vi "Check info str.vi"(8 "error in (no error)":errorcluster, 10 "Data in":string, 11 "Motor info":T1={"Motor positions"=[0.0, 0.0], "Sensor value"=0.0, "Ens-stop state"=[FALSE, FALSE], "°/step"=[], "Motor params"={"Action"=2, "Direction motor 1"=1, "Direction motor 2"=1, "Steps motor 1"=100, "Steps motor 2"=100, "Step style motor 1"=1, "Step style motor 2"=1}} {"Motor params"."Step style motor 2" items=["", "Single", "Double", "Interleave", "Microstep"]; "Motor params"."Step style motor 1" items=["", "Single", "Double", "Interleave", "Microstep"]; "Motor params"."Direction motor 2" items=["", "Forward", "Backward"]; "Motor params"."Direction motor 1" items=["", "Forward", "Backward"]; "Motor params"."Action" items=["", "Initialize", "Move"]; "°/step" format="%#_13g"}) -> (0 "error out":errorcluster, 3 "Motor info out":T1={"Motor positions"=[0.0, 0.0], "Sensor value"=0.0, "Ens-stop state"=[FALSE, FALSE], "°/step"=[], "Motor params"={"Action"=2, "Direction motor 1"=1, "Direction motor 2"=1, "Steps motor 1"=100, "Steps motor 2"=100, "Step style motor 1"=1, "Step style motor 2"=1}} {"Motor params"."Step style motor 2" items=["", "Single", "Double", "Interleave", "Microstep"]; "Motor params"."Step style motor 1" items=["", "Single", "Double", "Interleave", "Microstep"]; "Motor params"."Direction motor 2" items=["", "Forward", "Backward"]; "Motor params"."Direction motor 1" items=["", "Forward", "Backward"]; "Motor params"."Action" items=["", "Initialize", "Move"]; "°/step" format="%#_13g"})   [LabVIEW 2020, in "Control de MaP.lvlib"]
uses:
  Control de MaP.lvlib
  Controls/Motor info.ctl
  Controls/Move motor parameters--cluster.ctl
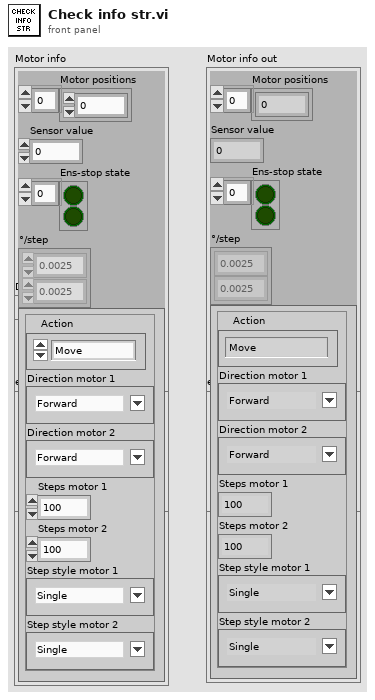
[diagram p1: front panel]
types:
  T1 = typedef "Control de MaP.lvlib/Motor info.ctl" = cluster{"Motor positions":dbl[], "Sensor value":dbl, "Ens-stop state":bool[], "°/step":dbl[], "Motor params":T2}
  T2 = typedef "Control de MaP.lvlib/Move motor parameters--cluster.ctl" = cluster{"Action":u8, "Direction motor 1":u8, "Direction motor 2":u8, "Steps motor 1":u16, "Steps motor 2":u16, "Step style motor 1":u8, "Step style motor 2":u8}
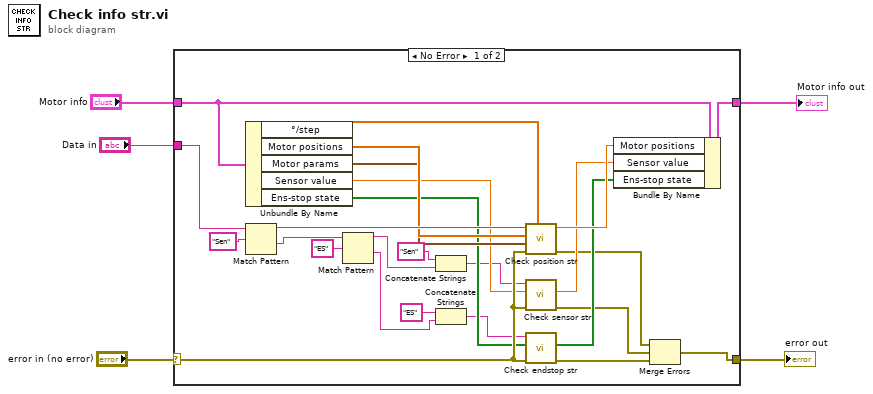
[diagram p0: block diagram]
diagram:
  n1 = case shown="No Error" "error in (no error)" {
    selector: "error in (no error)" -> [w21 w33]
    tunnel: "Data in" -> [w28 _]
    tunnel: [w17 w33] -> w3
    tunnel: "Motor info" -> [w25 w32]
    tunnel: [w15 w32] -> w1
    frame No Error {
      n2 = Unbundle By Name(w25) -> ("°/step"=w16:dbl[], "Motor positions"=w26:dbl[], "Motor params"=w14:T2, "Sensor value"=w13:dbl, "Ens-stop state"=w12:bool[])
      n3 = Match Pattern(string=w28, regular expression="Sen") -> (before substring=w27:string, after substring=w30:string)  [unwired: 1 in, 2 out]
      n4 = Match Pattern(string=w30, regular expression="ES") -> (before substring=w11:string, after substring=w7:string)  [unwired: 1 in, 2 out]
      n5 = Concatenate Strings("Sen" ("string"), w11) -> (w9:string)
      n6 = Concatenate Strings("ES" ("string"), w7) -> (w6:string)
      n7 = call "Check position str.vi"("mm/step"=w16, "error in (no error)"=w21, "Motor params"=w14, "Position in"=w26, "Recibo de Datos"=w27) -> ("error out"=w20:errorcluster, "Position out"=w24:dbl)  [unwired: 4 in, 1 out]
      n8 = call "Check sensor str.vi"("error in (no error)"=w21, "Sensor value in"=w13, "string"=w9) -> ("error out"=w19:errorcluster, "Sensor value out"=w23:dbl)  [unwired: 6 in]
      n9 = call "Check endstop str.vi"("error in (no error)"=w21, "Ens-stop state in"=w12, "Data in"=w6) -> ("error out"=w18:errorcluster, "Ens-stop state out"=w22:bool[])  [unwired: 7 in]
      n10 = Bundle By Name(cluster=w25, "Motor positions"=w24, "Sensor value"=w23, "Ens-stop state"=w22) -> (w15:T1)
      n11 = Merge Errors(w20, w19, w18) -> (w17:errorcluster)
    }
    frame Error {
    }
  }
  "error out" <- w3
  "Motor info out" <- w1
